vi "FMV - set cluster element.vi"(8 "error in (no error)":errorcluster, 11 "JSON string":string) -> (0 "error out":errorcluster, 3 "value":string)   [LabVIEW 2020, in "ui-testing.lvlib"]
doc: "copyright: Thomas Zilliox©"
uses:
  ui-testing.lvlib
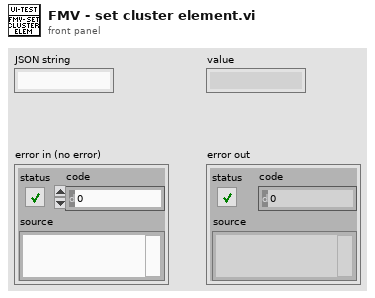
[diagram p1: front panel]
types:
  T1 = cluster{"name":string, "type":string, "value":string, "layers":string[]}
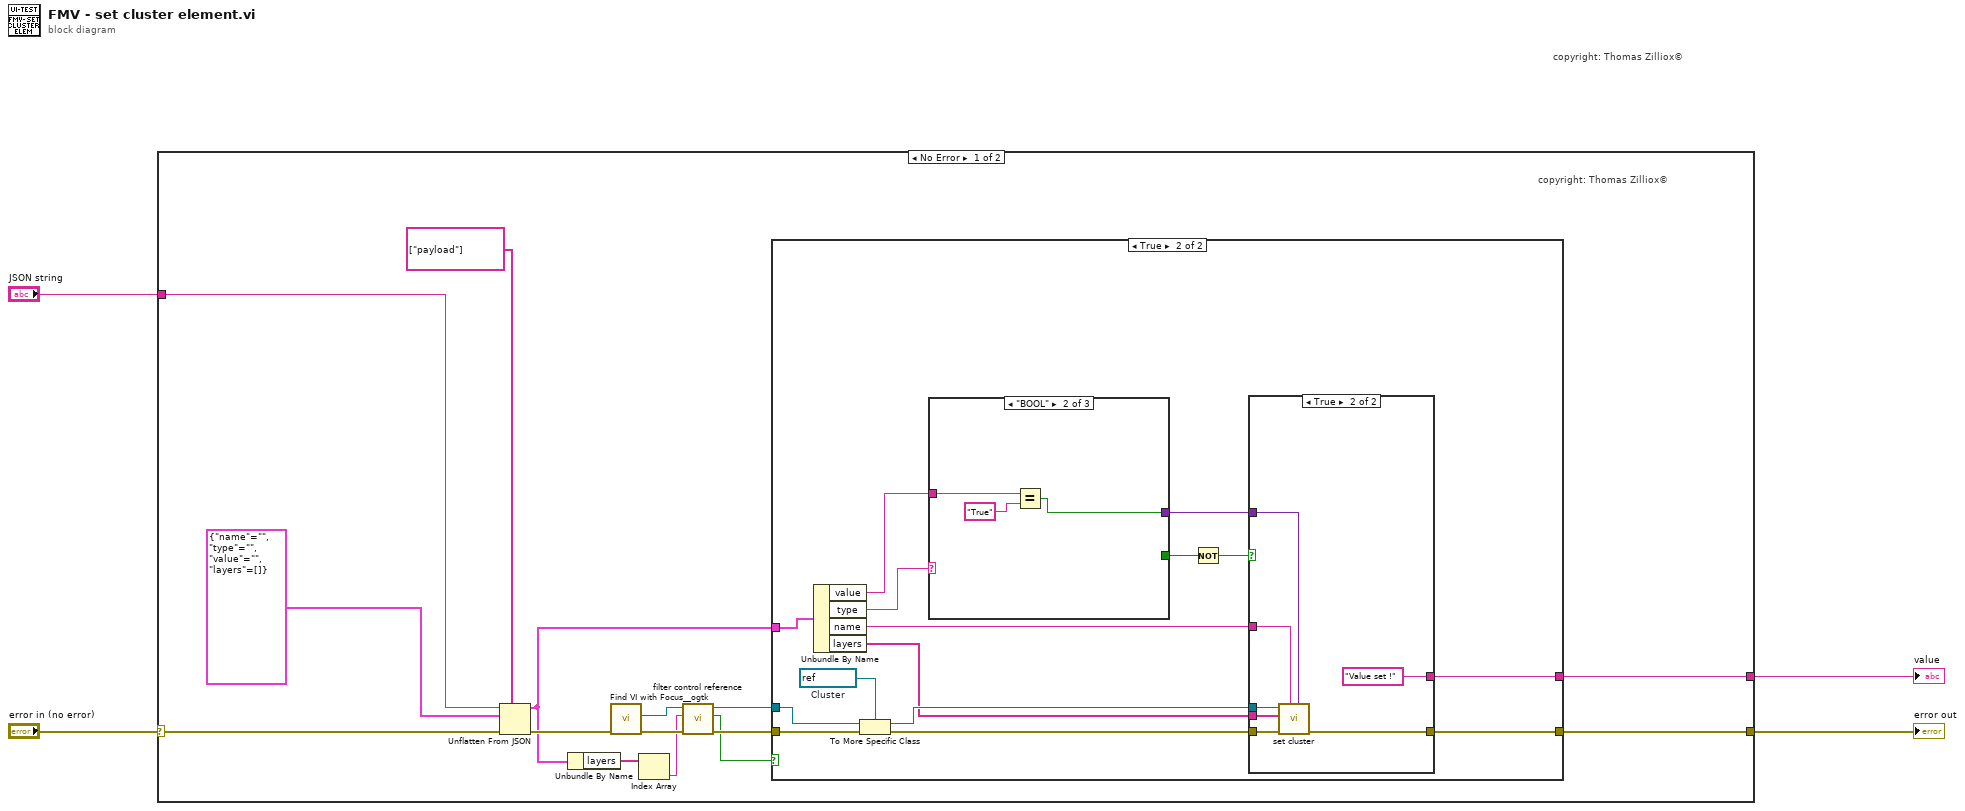
[diagram p0: block diagram]
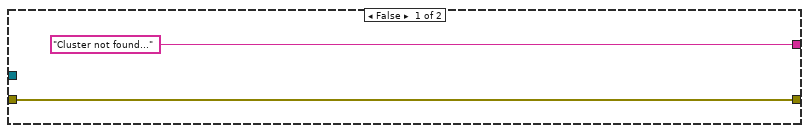
[diagram p2: hidden frame]
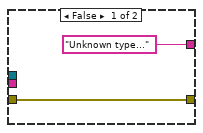
[diagram p3: hidden frame]
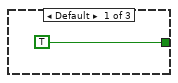
[diagram p4: hidden frame]
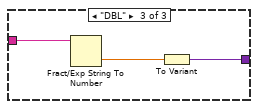
[diagram p5: hidden frame]
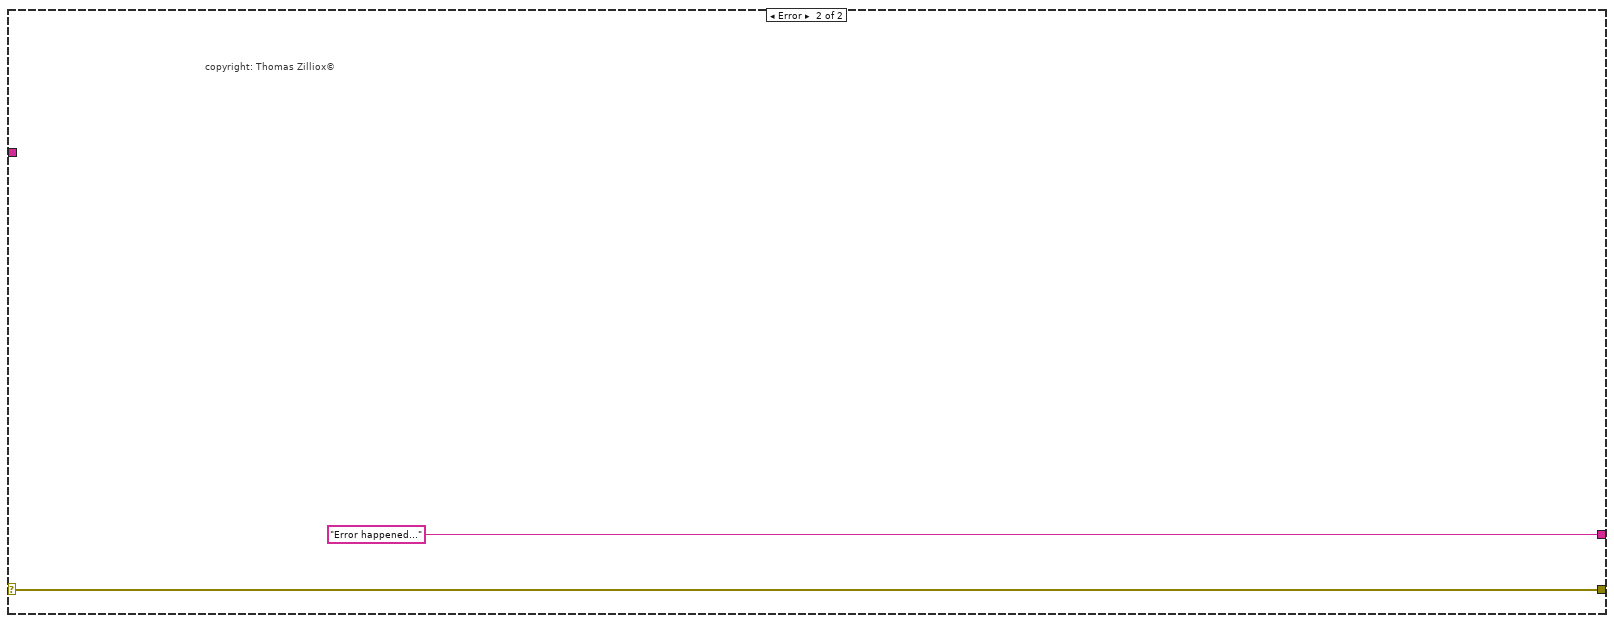
[diagram p6: hidden frame]
diagram:
  # "copyright: Thomas Zilliox©"
  n1 = case shown="No Error" "error in (no error)" {
    selector: "error in (no error)" -> [w17 w54]
    tunnel: "JSON string" -> [w18 _]
    tunnel: [w6 w54] -> w3
    tunnel: [w7 "Error happened..."] -> w2
    frame No Error {
      # "copyright: Thomas Zilliox©"
      n2 = Unflatten From JSON(path=string[] ["payload"], JSON string=w18, type and defaults=T1 {"name"="", "type"="", "value"="", "layers"=[]}, error in (no error)=w17) -> (value=w5:T1, error out=w16:errorcluster)  [unwired: 3 in]
      n3 = Unbundle By Name(w5) -> ("layers"=w12:string[])
      n4 = call <userlib>:"Find VI with Focus__ogtk.vi"("error in"=w16) -> ("error out"=w14:errorcluster, "VI with Focus"=w13:refnum<vi>)  [unwired: 6 in, 3 out]
      n5 = Index Array(array=w12) -> (element=w11:string)  [unwired: 1 in]
      n6 = call "filter control reference.vi"("error in (no error)"=w14, "Control label"=w11, "VI (Caller)"=w13) -> ("error out"=w9:errorcluster, "Control found"=w8:bool, "Control ref"=w10:refnum<vi>)  [unwired: 6 in]
      n7 = case shown="True" w8 {
        tunnel: w10 -> [_ w33]
        tunnel: w9 -> [w21 w36]
        tunnel: [w21 w35] -> w6
        tunnel: ["Cluster not found..." w24] -> w7
        tunnel: w5 -> [_ w30]
        frame False {
        }
        frame True {
          w31 = refnum<vi> refnum  # Cluster
          n8 = Unbundle By Name(w30) -> ("value"=w23:string, "type"=w27:string, "name"=w28:string, "layers"=w29:string[])
          n9 = To More Specific Class(target class=w31, reference=w33, error in=w36) -> (specific class reference=w32:refnum<vi>, error out=w34:errorcluster)
          n10 = case shown="\"BOOL\"" w27 {
            tunnel: [TRUE _ _] -> w26
            tunnel: [_ w47 w52] -> w22
            tunnel: w23 -> [_ w49 w51]
            frame Default {
            }
            frame "BOOL" {
              n11 = Equal?(x=w49, y="True") -> (x = y?=w47:bool)
            }
            frame "DBL" {
              n12 = Fract/Exp String To Number(string=w51) -> (number=w50:dbl)  [unwired: 3 in, 1 out]
              n13 = To Variant(anything=w50) -> (Variant=w52:variant)
            }
          }
          n14 = Not(x=w26) -> (.not. x?=w25:bool)
          n15 = case shown="True" w25 {
            tunnel: [w38 w45] -> w35
            tunnel: w34 -> [w38 w44]
            tunnel: w32 -> [_ w43]
            tunnel: w29 -> [_ w42]
            tunnel: w28 -> [_ w41]
            tunnel: ["Unknown type..." "Value set !"] -> w24
            tunnel: w22 -> [_ w39]
            frame False {
            }
            frame True {
              n16 = call "set cluster.vi"("Value"=w39, "Label"=w41, "error in (no error)"=w44, "Layer arrary"=w42, "cluster ref"=w43) -> ("error out"=w45:errorcluster)  [unwired: 6 in]
            }
          }
        }
      }
    }
    frame Error {
      # "copyright: Thomas Zilliox©"
    }
  }
  "error out" <- w3
  "value" <- w2
